vi "swiches.vi"(6 "Numeric 2":i16, 7 "Numeric":i16, 9 "Numeric 3":i16, 10 "Numeric 4":i16, 11 "Numeric 5":i16) -> (1 "xLength":dbl, 3 "yLength":dbl)   [LabVIEW 2017]
uses:
  Global pulses.vi
panel:
  out "Enum":T1(ring)
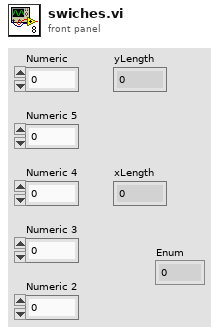
[diagram p1: front panel]
types:
  T1 = enum16{"0", "1", "2", "3", "4", "5", "6", "7", "8", "9", "10", "11"}
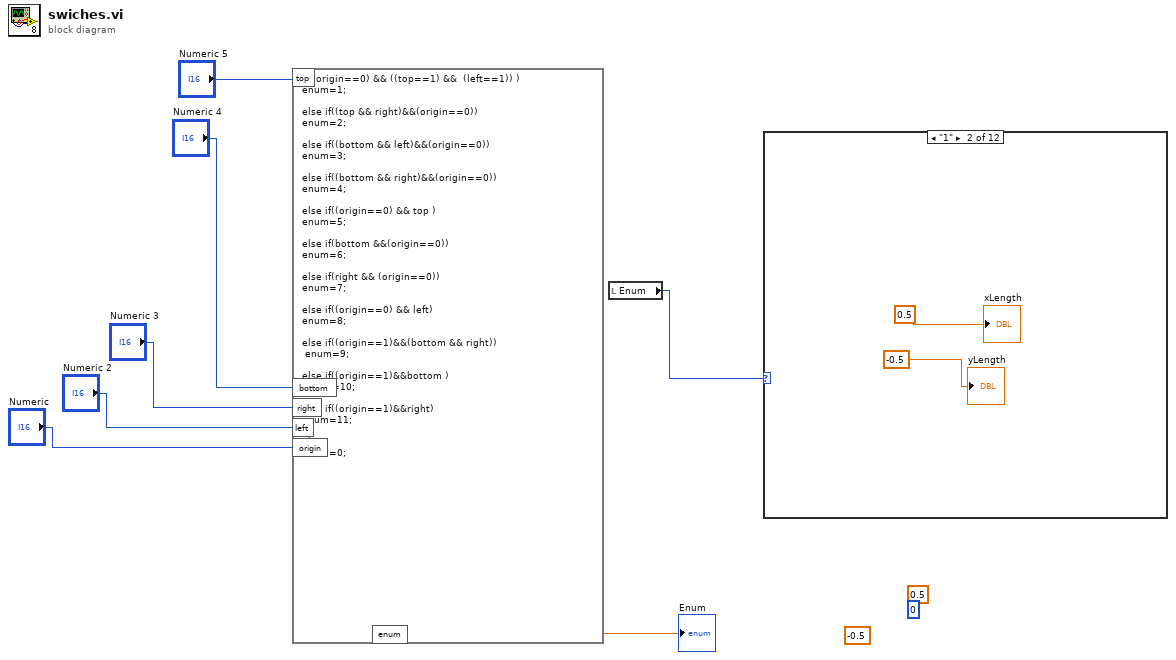
[diagram p0: block diagram]
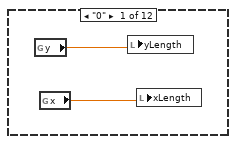
[diagram p2: hidden frame]
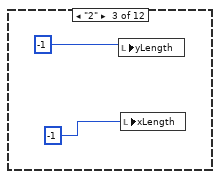
[diagram p3: hidden frame]
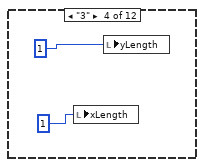
[diagram p4: hidden frame]
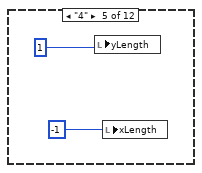
[diagram p5: hidden frame]
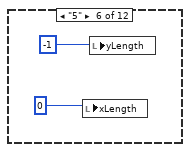
[diagram p6: hidden frame]
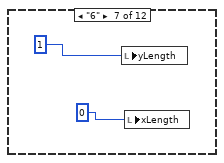
[diagram p7: hidden frame]
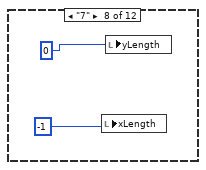
[diagram p8: hidden frame]
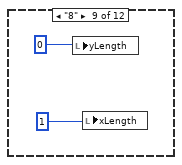
[diagram p9: hidden frame]
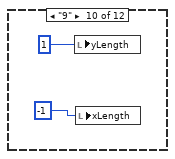
[diagram p10: hidden frame]
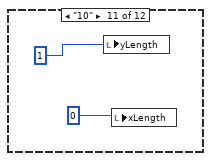
[diagram p11: hidden frame]
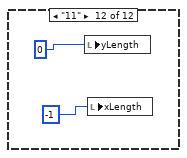
[diagram p12: hidden frame]
diagram:
  (unwired) 0.5
  (unwired) 0
  (unwired) -0.5
  n1 = formula code="if((origin==0) && ((top==1) &&  (left==1)) )\nenum=1;\n\nelse if((top && right)&&(origin==0))\nenum=2;\n\nelse if((bottom && left)&&(origin==0))\nenum=3;\n\nelse if((bottom && right)&&(origin==0))\nenum=4;\n\nelse if((origin==0) && top )\nenum=5;\n\nelse if(bottom &&(origin==0))\nenum=6;\n\nelse if(right && (origin==0))\nenum=7;\n\nelse if((origin==0) && left)\nenum=8;\n\nelse if((origin==1)&&(bottom && right))\n enum=9;\n\nelse if((origin==1)&&bottom )\n enum=10;\n\nelse if((origin==1)&&right)\nenum=11;\n\nelse\nenum=0;"("top"="Numeric 5", "bottom"="Numeric 4", "right"="Numeric 3", "left"="Numeric 2", "origin"="Numeric") -> ("enum"=→"Enum":dbl)
  n2 = local read "Enum"() -> (w1:T1)
  n3 = case shown="\"1\"" w1 {
    frame "0" {
      n4 = global read "Global pulses.vi" "y"() -> (w9:dbl)
      n5 = global read "Global pulses.vi" "x"() -> (w8:dbl)
      n6 = local write "yLength"(w9) -> ()
      n7 = local write "xLength"(w8) -> ()
    }
    frame "1" {
      "xLength" <- 0.5
      "yLength" <- -0.5
    }
    frame "2" {
      n8 = local write "yLength"(-1) -> ()
      n9 = local write "xLength"(-1) -> ()
    }
    frame "3" {
      n10 = local write "xLength"(1) -> ()
      n11 = local write "yLength"(1) -> ()
    }
    frame "4" {
      n12 = local write "yLength"(1) -> ()
      n13 = local write "xLength"(-1) -> ()
    }
    frame "5" {
      n14 = local write "xLength"(0) -> ()
      n15 = local write "yLength"(-1) -> ()
    }
    frame "6" {
      n16 = local write "yLength"(1) -> ()
      n17 = local write "xLength"(0) -> ()
    }
    frame "7" {
      n18 = local write "xLength"(-1) -> ()
      n19 = local write "yLength"(0) -> ()
    }
    frame "8" {
      n20 = local write "yLength"(0) -> ()
      n21 = local write "xLength"(1) -> ()
    }
    frame "9" {
      n22 = local write "yLength"(1) -> ()
      n23 = local write "xLength"(-1) -> ()
    }
    frame "10" {
      n24 = local write "yLength"(1) -> ()
      n25 = local write "xLength"(0) -> ()
    }
    frame "11" {
      n26 = local write "yLength"(0) -> ()
      n27 = local write "xLength"(-1) -> ()
    }
  }
